vi "RS232 Read Integer.vi"(0 "Setup in":T6={"No.VI"=0, "Category"="", "StepName"="", "Seq setup flattened"="", "Comment"="", "Steps config."=[], "Jump config"=[], "Start"=0.0, "Increment"=0.0, "Name"="Pa", "Unit"="Pa", "Y data"=1, "Y prefix"="", "Y dB ref"=1.0, "Y unit"="", "Repeat State Array"=[]} {"Repeat State Array"."Start" format="%#_5g"; "Y dB ref" format="%.1f"; "Y data" items=["dB", "Lin"]; "Start" format="%#_5g"}, 5 "Data in":T4 {"Z data" items=["dB", "Lin"]; "X data" items=["dB", "Lin"]; "Y data" items=["dB", "Lin"]; "Z dB ref" format="%.1f"; "Z axis" items=["Log", "Lin"]; "X dB ref" format="%.1f"; "X axis" items=["Log", "Lin"]; "Y axis" items=["Log", "Lin"]; "Y dB ref" format="%.1f"; "Curve"."z" format="%.2f"; "Curve"."y" format="%.2f"; "Curve"."x" format="%.2f"}, 7 "Results in":T2 {"Margin" format="%.2f"}, 9 "Seq Setup in":string, 11 "Step name":string, 12 "Hardware in":string, 13 "Calibration in":string) -> (3 "Types Out":string[](array[string]), 4 "Inserted Names Out":string[](array[string]), 6 "Data out":T4 {"Z data" items=["dB", "Lin"]; "X data" items=["dB", "Lin"]; "Y data" items=["dB", "Lin"]; "Z dB ref" format="%.1f"; "Z axis" items=["Log", "Lin"]; "X dB ref" format="%.1f"; "X axis" items=["Log", "Lin"]; "Y axis" items=["Log", "Lin"]; "Y dB ref" format="%.1f"; "Curve"."z" format="%.2f"; "Curve"."y" format="%.2f"; "Curve"."x" format="%.2f"}, 8 "Results out":T2 {"Margin" format="%.2f"}, 10 "Wave out":T1[](array[typedef]) {"Y dB ref" format="%.1f"; "Y axis" items=["Log", "Lin"]; "Y data" items=["dB", "Lin"]; "X data" items=["dB", "Lin"]})   [LabVIEW 2013]
uses:
  CRYCustom and Run Seq.llb/CRYData Cluster Array.ctl
  CRYCustom and Run Seq.llb/CRYData Cluster.ctl
  CRYCustom and Run Seq.llb/CRYResult Cluster Array.ctl
  CRYCustom and Run Seq.llb/CRYResult Cluster.ctl
  CRYCustom and Run Seq.llb/CRYStep.ctl
  CRYCustom and Run Seq.llb/CRYWaveform Cluster.ctl
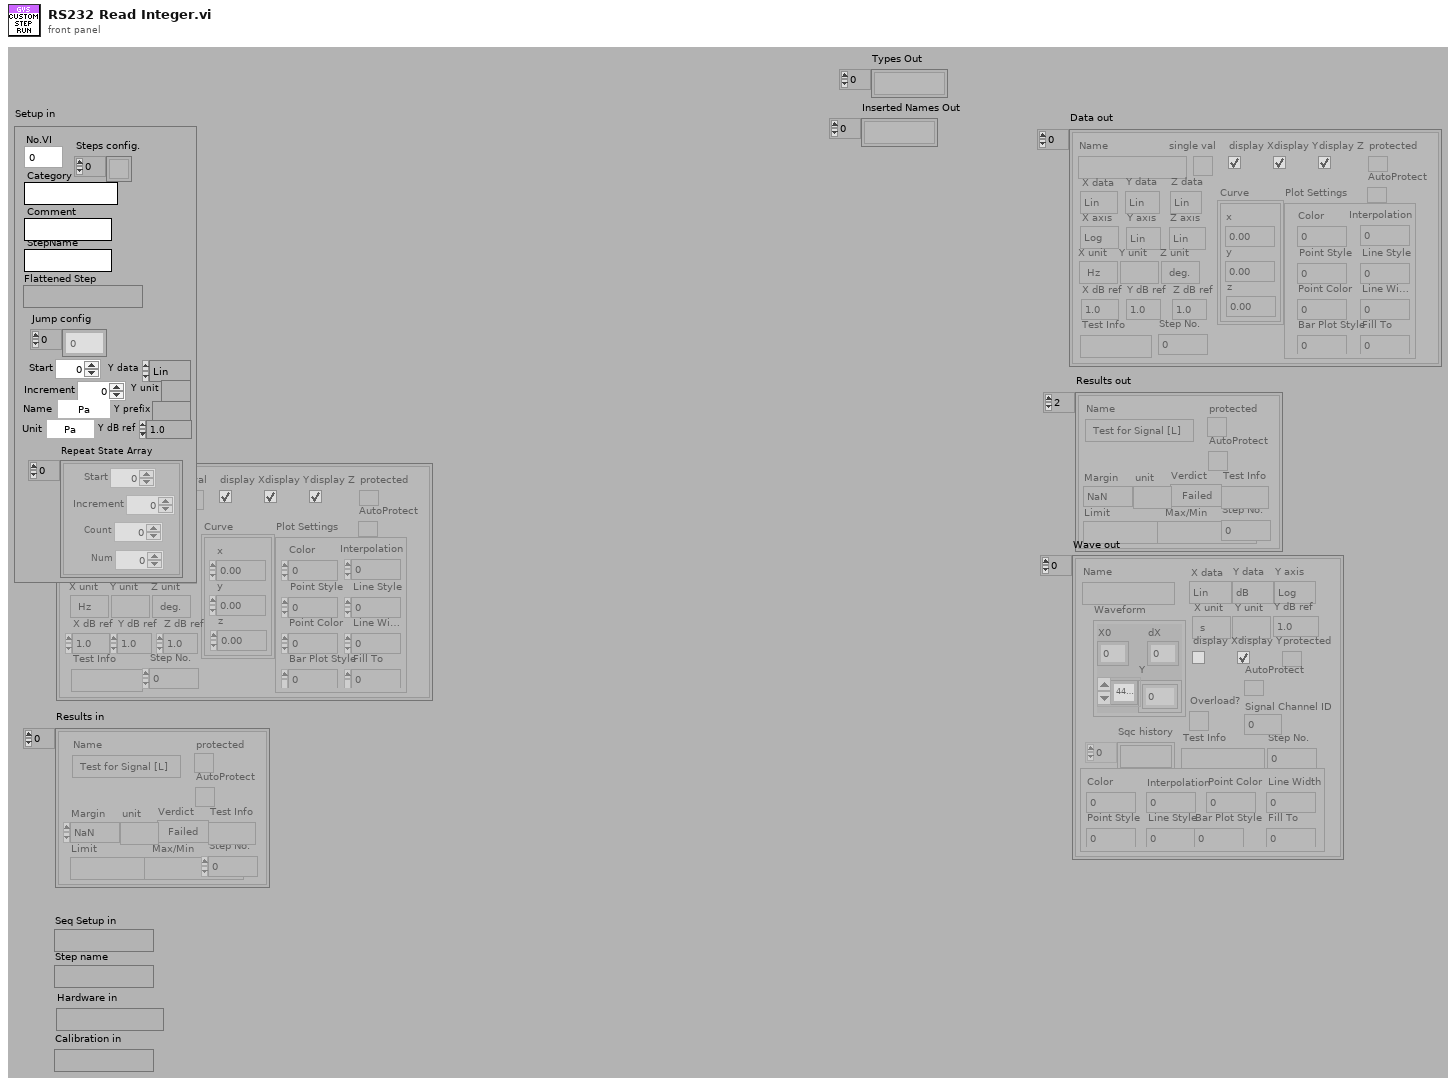
[diagram p1: front panel]
types:
  T1 = typedef "CRYWaveform Cluster.ctl" = cluster{"Waveform":cluster{"X0":dbl, "dX":dbl, "Y":sgl[]}, "X data":u16, "Y data":u16, "Y axis":u16, "X unit":string, "Y unit":string, "Y dB ref":dbl, "display Y":bool, "display X":bool, "Overload?":bool, "Test Info":string, "Step No.":i32, "Name":string, "protected":bool, "Sqc history":string[], "Signal Channel ID":i32, "Plot Settings":cluster{"Color":u32, "Interpolation":u8, "Point Style":u8, "Line Style":u8, "Point Color":u32, "Line Width":u8, "Bar Plot Style":u8, "Fill To":i16}, "AutoProtect":bool}
  T2 = typedef "CRYResult Cluster Array.ctl" = T3[]
  T3 = typedef "CRYResult Cluster.ctl" = cluster{"Name":string, "Margin":dbl, "unit":string, "Verdict":bool, "Limit":string, "Max/Min":string, "protected":bool, "Step No.":i32, "Test Info":string, "AutoProtect":bool}
  T4 = typedef "CRYData Cluster Array.ctl" = T5[]
  T5 = typedef "CRYData Cluster.ctl" = cluster{"Name":string, "Curve":cluster{"x":dbl, "y":dbl, "z":dbl}[], "X data":u16, "Y data":u16, "Z data":u16, "X axis":u16, "Y axis":u16, "Z axis":u16, "X unit":string, "Y unit":string, "Z unit":string, "X dB ref":dbl, "Y dB ref":dbl, "Z dB ref":dbl, "single val":bool, "protected":bool, "display X":bool, "display Y":bool, "display Z":bool, "Test Info":string, "Step No.":i32, "Plot Settings":cluster{"Color":u32, "Interpolation":u8, "Point Style":u8, "Line Style":u8, "Point Color":u32, "Line Width":u8, "Bar Plot Style":u8, "Fill To":i16}, "AutoProtect":bool}
  T6 = typedef "CRYStep.ctl" = cluster{"No.VI":i32, "Category":string, "StepName":string, "Seq setup flattened":string, "Comment":string, "Steps config.":bool[], "Jump config":i32[], "Start":dbl, "Increment":dbl, "Name":string, "Unit":string, "Y data":u16, "Y prefix":string, "Y dB ref":dbl, "Y unit":string, "Repeat State Array":cluster{"Start":dbl, "Increment":dbl, "Count":i32, "Num":i32}[]}
  T7 = cluster{"Type":u16, "Select COM Port":i32, "Byte":i32, "Unit":string, "Curve Name":string}
  T8 = typedef "CRYCustom Cluster.ctl" = cluster{"Help":string, "Flatten Data":string}
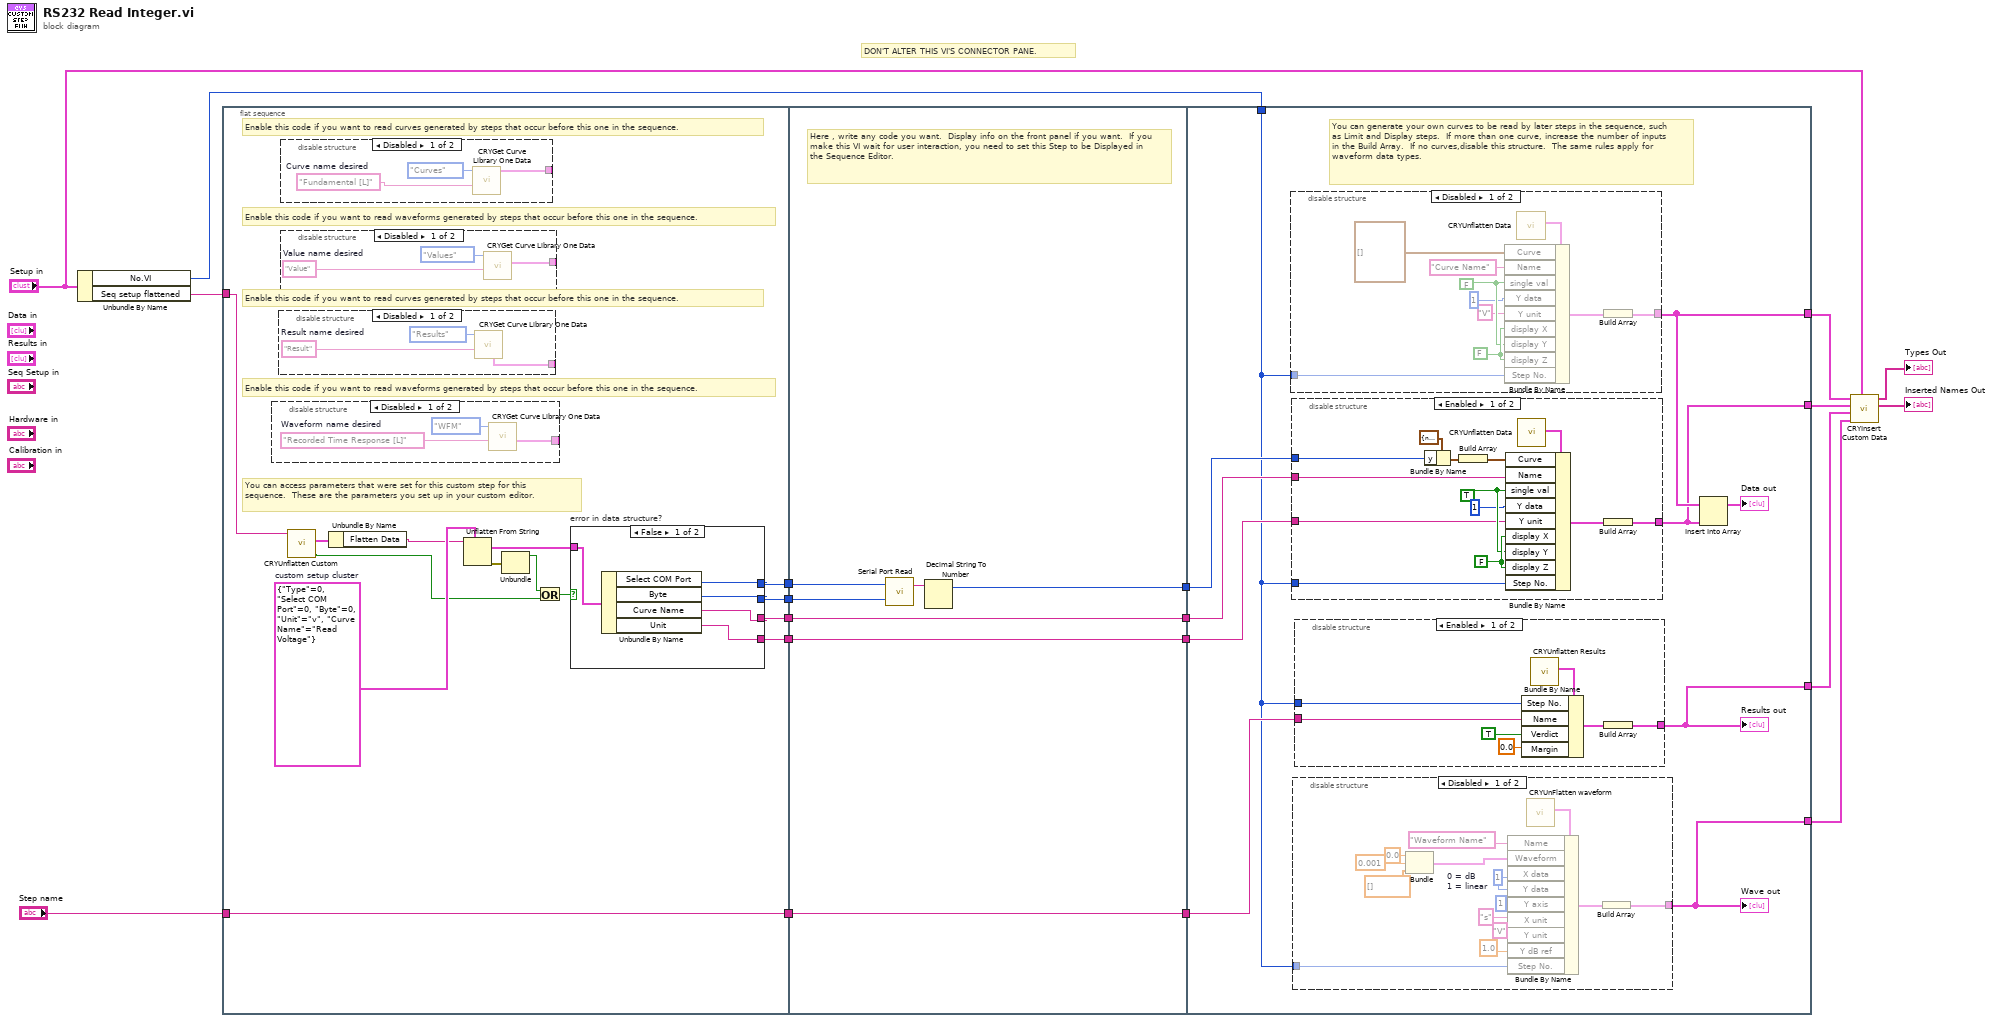
[diagram p0: block diagram]
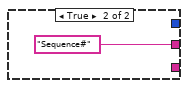
[diagram p6: hidden frame]
diagram:
  # "DON'T ALTER THIS VI'S CONNECTOR PANE."
  n1 = Unbundle By Name("Setup in") -> ("No.VI"=w8:i32, "Seq setup flattened"=w19:string)
  n2 = flat-sequence {
    tunnel: w19 -> [w22]
    tunnel: "Step name" -> [w24]
    tunnel: [w28] -> w17
    tunnel: [w27] -> w16
    tunnel: [w26] -> w15
    tunnel: [w25] -> w14
    tunnel: [w24] -> w13
    tunnel: w17 -> [w58]
    tunnel: w16 -> [w57]
    tunnel: w15 -> [w54]
    tunnel: w14 -> [w53]
    tunnel: w13 -> [w56]
    tunnel: [w58] -> w12
    tunnel: [w57] -> w11
    tunnel: [w56] -> w10
    tunnel: [w52] -> w9
    tunnel: w12 -> [w68]
    tunnel: w11 -> [w65]
    tunnel: w10 -> [w67]
    tunnel: w9 -> [w63]
    tunnel: [w66] -> w5
    tunnel: [w60] -> w6
    tunnel: w8 -> [w62]
    tunnel: [w64] -> w4
    tunnel: [w61] -> w7
    frame #0 {
      w29 = T7 {"Type"=0, "Select COM Port"=0, "Byte"=0, "Unit"="v", "Curve Name"="Read Voltage"}  # custom setup cluster
      # "Enable this code if you want to read waveforms generated by steps that occur before this one in the sequence."
      # "Enable this code if you want to read curves generated by steps that occur before this one in the sequence."
      # "Enable this code if you want to read waveforms generated by steps that occur before this one in the sequence."
      # "Enable this code if you want to read curves generated by steps that occur before this one in the sequence."
      # "You can access parameters that were set for this custom step for this sequence.  These are the parameters you set up in your custom editor."
      n3 = disable-structure shown="Disabled" {
        disable-tunnel: [w38 _] -> _
        frame Disabled {
          w37 = "Recorded Time Response [L]"  # Waveform name desired
          n4 = call "CRYGet Curve Library One Data .vi"("Data Name"=w37, "Type"=enum16{"Curves", "Values", "Results", "WFM"}."WFM") -> ("Wave"=w38:T1)  [unwired: 3 in, 6 out]
        }
        frame Enabled {
        }
      }
      n5 = disable-structure shown="Disabled" {
        disable-tunnel: [w34 _] -> _
        frame Disabled {
          w35 = "Result"  # Result name desired
          n6 = call "CRYGet Curve Library One Data .vi"("Data Name"=w35, "Type"=enum16{"Curves", "Values", "Results", "WFM"}."Results") -> ("Result"=w34:T3)  [unwired: 3 in, 6 out]
        }
        frame Enabled {
        }
      }
      n7 = disable-structure shown="Disabled" {
        disable-tunnel: [w40 _] -> _
        frame Disabled {
          w41 = "Fundamental [L]"  # Curve name desired
          n8 = call "CRYGet Curve Library One Data .vi"("Data Name"=w41, "Type"=enum16{"Curves", "Values", "Results", "WFM"}."Curves") -> ("Curve"=w40:T5)  [unwired: 3 in, 6 out]
        }
        frame Enabled {
        }
      }
      n9 = disable-structure shown="Disabled" {
        disable-tunnel: [w43 _] -> _
        frame Disabled {
          w44 = "Value"  # Value name desired
          n10 = call "CRYGet Curve Library One Data .vi"("Data Name"=w44, "Type"=enum16{"Curves", "Values", "Results", "WFM"}."Values") -> ("Value"=w43:T5)  [unwired: 3 in, 6 out]
        }
        frame Enabled {
        }
      }
      n11 = call "CRYUnflatten Custom.vi"("Unflatten Custom"=w22) -> ("Error?"=w21:bool, "Custom"=w23:T8)  [unwired: 8 in, 1 out]
      n12 = Unbundle By Name(w23) -> ("Flatten Data"=w20:string)
      n13 = Unflatten From String(type=w29, binary string=w20) -> (value=w32:T7, error out=w33:errorcluster)  [unwired: 1 in, 3 out]
      n14 = Unbundle(w33) -> ("status"=w30:bool)  [unwired: 2 out]
      n15 = Or(x=w30, y=w21) -> (x .or. y?=w31:bool)
      n16 = case "error in data structure?" shown="False" w31 {
        tunnel: w32 -> [w50 _]
        tunnel: [w46 _] -> w25
        tunnel: [w49 "Sequence#" ("Name")] -> w28
        tunnel: [w48 _] -> w27
        tunnel: [w47 _] -> w26
        frame False {
          n17 = Unbundle By Name(w50) -> ("Select COM Port"=w47:i32, "Byte"=w46:i32, "Curve Name"=w49:string, "Unit"=w48:string)
        }
        frame True {
        }
      }
    }
    frame #1 {
      # "Here , write any code you want.  Display info on the front panel if you want.  If you make this VI wait for user interaction, you need to set this Step to be Displayed in the Sequence Editor."
      n18 = call <vilib>:"Serial Port Read.vi"("requested byte count"=w53, "port number"=w54) -> ("string read"=w55:string)  [unwired: 1 out]
      n19 = Decimal String To Number(string=w55) -> (offset past number=w52:i32)  [unwired: 2 in, 1 out]
    }
    frame #2 {
      # "You can generate your own curves to be read by later steps in the sequence, such as Limit and Display steps.  If more than one curve, increase the number of inputs in the Build Array.  If no curves,disable this structure.  The same rules apply for waveform data types."
      n20 = disable-structure shown="Disabled" {
        disable-tunnel: w62 -> [w74 _]
        disable-tunnel: [w69 _] -> w61
        frame Disabled {
          w77 = FALSE
          w76 = FALSE
          n21 = call "CRYUnflatten Data.vi"() -> ("Datum"=w78:T5)  [unwired: 9 in, 2 out]
          n22 = Bundle By Name(cluster=w78, "Curve"=cluster{"x":dbl, "y":dbl, "z":dbl}[] [] ("appended array"), "Name"="Curve Name", "single val"=w76, "Y data"=u16 1, "Y unit"="V", "display X"=w77, "display Y"=w76, "display Z"=w77, "Step No."=w74) -> (w70:T5)
          n23 = Build Array(w70) -> (w69:T5[])
        }
        frame Enabled {
        }
      }
      n24 = disable-structure shown="Enabled" {
        disable-tunnel: w62 -> [w84 _]
        disable-tunnel: w63 -> [w83 _]
        disable-tunnel: w68 -> [w82 _]
        disable-tunnel: w65 -> [w81 _]
        disable-tunnel: [w79 _] -> w60
        frame Enabled {
          w87 = FALSE
          w86 = TRUE
          n25 = Bundle By Name(cluster=cluster{"x":dbl, "y":dbl, "z":dbl} {"x"=nan, "y"=0.0, "z"=nan}, "y"=w83) -> (w89:cluster{"x":dbl, "y":dbl, "z":dbl})
          n26 = Build Array(w89) -> (w90:cluster{"x":dbl, "y":dbl, "z":dbl}[])
          n27 = call "CRYUnflatten Data.vi"() -> ("Datum"=w91:T5)  [unwired: 9 in, 2 out]
          n28 = Bundle By Name(cluster=w91, "Curve"=w90, "Name"=w82, "single val"=w86, "Y data"=u16 1, "Y unit"=w81, "display X"=w87, "display Y"=w86, "display Z"=w87, "Step No."=w84) -> (w80:T5)
          n29 = Build Array(w80) -> (w79:T5[])
        }
        frame Disabled {
        }
      }
      n30 = disable-structure shown="Disabled" {
        disable-tunnel: [w100 _] -> w64
        disable-tunnel: w62 -> [w99 _]
        frame Disabled {
          w105 = u16 1  # 0 = dB 1 = linear
          n31 = Bundle ("Actual waveform data bundle.\nX0\ndX\n[Y] array")(0.0, 0.001, dbl[] []) -> (w109:cluster{dbl, dbl, dbl[]})  [unwired: 1 out]
          n32 = call "CRYUnFlatten waveform.vi"() -> ("Waveform Cluster"=w110:T1)  [unwired: 9 in, 2 out]
          n33 = Bundle By Name(cluster=w110, "Name"="Waveform Name" ("Bundle Element"), "Waveform"=w109, "X data"=w105, "Y data"=w105, "Y axis"=u16 1, "X unit"="s", "Y unit"="V", "Y dB ref"=1.0, "Step No."=w99) -> (w111:T1)
          n34 = Build Array(w111) -> (w100:T1[])
        }
        frame Enabled {
        }
      }
      "Wave out" <- w64
      n35 = disable-structure shown="Enabled" {
        disable-tunnel: w62 -> [w94 _]
        disable-tunnel: w67 -> [w93 _]
        disable-tunnel: [w92 _] -> w66
        frame Enabled {
          n36 = call "CRYUnflatten Results.vi"() -> ("Result"=w95:T3)  [unwired: 9 in, 2 out]
          n37 = Bundle By Name(cluster=w95, "Step No."=w94, "Name"=w93, "Verdict"=TRUE, "Margin"=0.0) -> (w97:T3)
          n38 = Build Array(w97) -> (w92:T3[])
        }
        frame Disabled {
        }
      }
      "Results out" <- w66
      n39 = Insert Into Array(array=w61, new element=w60) -> (→"Data out":T5[])  [unwired: 1 in]
    }
  }
  n40 = call "CRYInsert Custom Data.vi"("Setup in"="Setup in", "Wave"=w4, "Results"=w5, "Values"=w6, "Curves"=w7) -> ("Inserted Names Out"=→"Inserted Names Out":string[], "Types Out"=→"Types Out":string[])  [unwired: 5 in]
